vi "Deserialize File Attributes.vi"(8 "error in":errorcluster, 11 "packet":u8[](array[numeric])) -> (0 "error out":errorcluster, 2 "file attributes":T1 {"permissions" format="%04o"}, 3 "packet remaining":u8[](array[numeric]))   [LabVIEW 2020, in "NI_SFTP.lvlib"]
uses:
  <vilib>/net/SFTP/NI_SFTP.lvlib
  <vilib>/net/SFTP/API/Support/File Attributes.ctl
  d022a744-54a9-3fd3-903f-96656418eb3f.vi
  344b3680-f82e-3fd4-783f-4678d93fd33f.vi
  ad0e4a4c-18fc-3fe0-0060-795593d7b03f.vi
  adfa6818-b576-3fe4-a010-b17c7da7e73f.vi
  0b12cbf9-0ffd-3fec-4b35-d5464624ee3f.vi
  d1b708d0-cdb1-3fdd-e8ab-91f32da9d03f.vi
  8c3f788a-5d1b-3fe5-114b-6415c22bea3f.vi
  7090e118-4d07-3fef-a0e5-9088025bb73f.vi
  96fe2671-f19e-3fdc-e0fb-be93fff4e23f.vi
  d13a85d0-f59b-3fbc-06cd-154f57cdda3f.vi
  <vilib>/net/SFTP/Low Level Connection/Assert Length.vi
  <vilib>/Bit Manipulation/Network-Order Bytes To Words Poly.vi
  <vilib>/Bit Manipulation/wrappers/Network-Order Bytes To Words/Network-Order Bytes To Words U32.vi
  <vilib>/Bit Manipulation/wrappers/Network-Order Bytes To Words/Network-Order Bytes To Words U64.vi
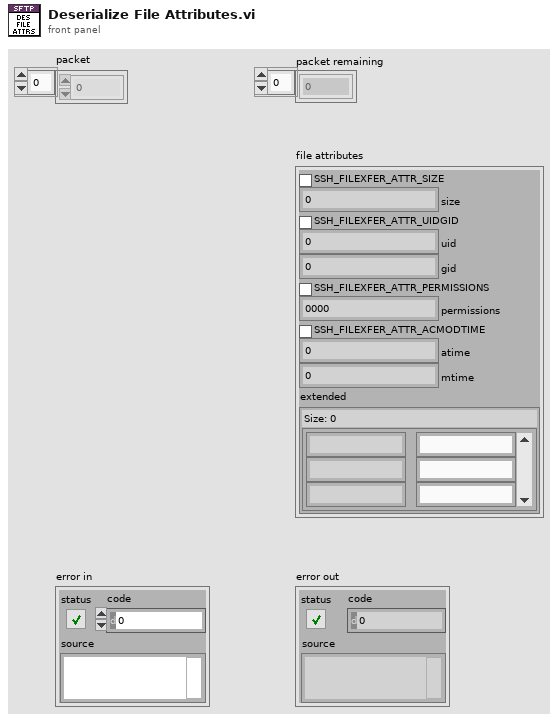
[diagram p1: front panel]
types:
  T1 = typedef "NI_SFTP.lvlib/File Attributes.ctl" = cluster{"SSH_FILEXFER_ATTR_SIZE":bool, "size":u64, "SSH_FILEXFER_ATTR_UIDGID":bool, "uid":u32, "gid":u32, "SSH_FILEXFER_ATTR_PERMISSIONS":bool, "permissions":u32, "SSH_FILEXFER_ATTR_ACMODTIME":bool, "atime":u32, "mtime":u32, "extended":map{string, string}}
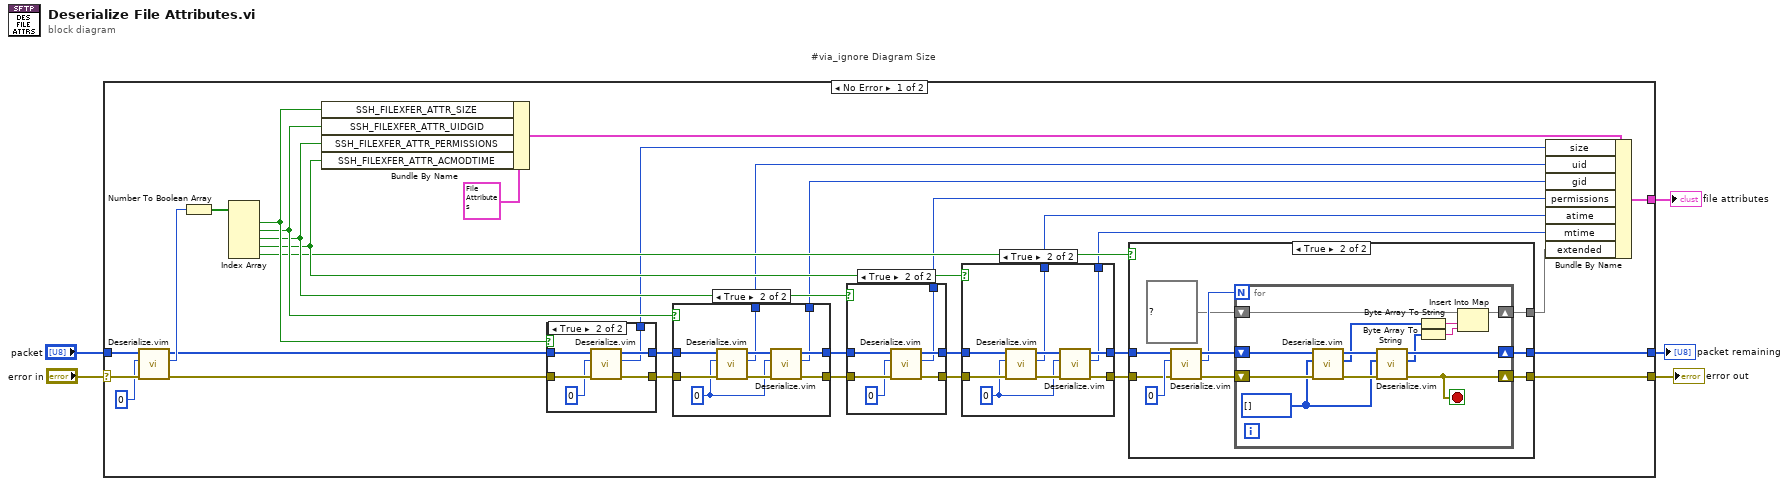
[diagram p0: block diagram]
diagram:
  # "#via_ignore Diagram Size"
  n1 = case shown="No Error" "error in" {
    selector: "error in" -> [w36 w102]
    tunnel: "packet" -> [w37 w101]
    tunnel: [w16 w102] -> w3
    tunnel: [w13 _] -> w2
    tunnel: [w15 w101] -> w1
    frame No Error {
      n2 = call "Deserialize.vim"("error in"=w36, "type"=u32 0, "bytes"=w37) -> ("error out"=w29:errorcluster, "value"=w34:u32, "remaining bytes"=w30:u8[])  [unwired: 6 in]
      n3 = Number To Boolean Array(number=w34) -> (Boolean array=w33:bool[])
      n4 = Index Array(array=w33) -> (element #1=w31:bool, element #2=w28:bool, element #3=w25:bool, element #4=w20:bool, element #5=w19:bool)  [unwired: 5 in]
      n5 = Bundle By Name(cluster=T1 {"SSH_FILEXFER_ATTR_SIZE"=FALSE, "size"=0, "SSH_FILEXFER_ATTR_UIDGID"=FALSE, "uid"=0, "gid"=0, "SSH_FILEXFER_ATTR_PERMISSIONS"=FALSE, "permissions"=0, "SSH_FILEXFER_ATTR_ACMODTIME"=FALSE, "atime"=0, "mtime"=0, "extended"={}} ("File Attributes"), "SSH_FILEXFER_ATTR_SIZE"=w31, "SSH_FILEXFER_ATTR_UIDGID"=w28, "SSH_FILEXFER_ATTR_PERMISSIONS"=w25, "SSH_FILEXFER_ATTR_ACMODTIME"=w20) -> (w6:T1)
      n6 = case shown="True" w31 {
        tunnel: w30 -> [w94 w100]
        tunnel: w29 -> [w93 w99]
        tunnel: [w94 w97] -> w27
        tunnel: [w93 w96] -> w26
        tunnel: [_ w95] -> w7
        frame False {
        }
        frame True {
          n7 = call "Deserialize.vim"("error in"=w99, "type"=u64 0, "bytes"=w100) -> ("error out"=w96:errorcluster, "value"=w95:u64, "remaining bytes"=w97:u8[])  [unwired: 6 in]
        }
      }
      n8 = case shown="True" w28 {
        tunnel: w27 -> [w83 w92]
        tunnel: w26 -> [w82 w91]
        tunnel: [w83 w87] -> w24
        tunnel: [w82 w86] -> w23
        tunnel: [_ w85] -> w9
        tunnel: [_ w84] -> w8
        frame False {
        }
        frame True {
          w88 = u32 0
          n9 = call "Deserialize.vim"("error in"=w91, "type"=w88, "bytes"=w92) -> ("error out"=w89:errorcluster, "value"=w85:u32, "remaining bytes"=w90:u8[])  [unwired: 6 in]
          n10 = call "Deserialize.vim"("error in"=w89, "type"=w88, "bytes"=w90) -> ("error out"=w86:errorcluster, "value"=w84:u32, "remaining bytes"=w87:u8[])  [unwired: 6 in]
        }
      }
      n11 = case shown="True" w25 {
        tunnel: w24 -> [w75 w81]
        tunnel: w23 -> [w74 w80]
        tunnel: [w75 w78] -> w22
        tunnel: [w74 w77] -> w21
        tunnel: [_ w76] -> w10
        frame False {
        }
        frame True {
          n12 = call "Deserialize.vim"("error in"=w80, "type"=u32 0, "bytes"=w81) -> ("error out"=w77:errorcluster, "value"=w76:u32, "remaining bytes"=w78:u8[])  [unwired: 6 in]
        }
      }
      n13 = case shown="True" w20 {
        tunnel: w22 -> [w64 w73]
        tunnel: w21 -> [w63 w72]
        tunnel: [w64 w68] -> w18
        tunnel: [w63 w67] -> w17
        tunnel: [_ w66] -> w12
        tunnel: [_ w65] -> w11
        frame False {
        }
        frame True {
          w69 = u32 0
          n14 = call "Deserialize.vim"("error in"=w72, "type"=w69, "bytes"=w73) -> ("error out"=w70:errorcluster, "value"=w66:u32, "remaining bytes"=w71:u8[])  [unwired: 6 in]
          n15 = call "Deserialize.vim"("error in"=w70, "type"=w69, "bytes"=w71) -> ("error out"=w67:errorcluster, "value"=w65:u32, "remaining bytes"=w68:u8[])  [unwired: 6 in]
        }
      }
      n16 = case shown="True" w19 {
        tunnel: w18 -> [w39 w48]
        tunnel: w17 -> [w38 w47]
        tunnel: [w39 w42] -> w15
        tunnel: [w38 w41] -> w16
        tunnel: [_ w40] -> w14
        frame False {
        }
        frame True {
          n17 = call "Deserialize.vim"("error in"=w47, "type"=u32 0, "bytes"=w48) -> ("error out"=w45:errorcluster, "value"=w44:u32, "remaining bytes"=w46:u8[])  [unwired: 6 in]
          n18 = for {
            N: w44 -> [_]
            shift-right: [w56] -> w42
            shift-left: w46 -> [w62]
            shift-right: [w55] -> w41
            shift-left: w45 -> [w61]
            shift-right: [w57] -> w40
            shift-left: map{string, string} {} ("extended") -> [w58]
            stop <- w55 stop-if-true
            w54 = u8[] [] ("Array")
            n19 = call "Deserialize.vim"("error in"=w61, "type"=w54, "bytes"=w62) -> ("error out"=w59:errorcluster, "value"=w53:u8[], "remaining bytes"=w60:u8[])  [unwired: 6 in]
            n20 = call "Deserialize.vim"("error in"=w59, "type"=w54, "bytes"=w60) -> ("error out"=w55:errorcluster, "value"=w51:u8[], "remaining bytes"=w56:u8[])  [unwired: 6 in]
            n21 = Byte Array To String(unsigned byte array=w53) -> (string=w52:string)
            n22 = Byte Array To String(unsigned byte array=w51) -> (string=w50:string)
            n23 = Insert Into Map(map in=w58, key=w52, value=w50) -> (map out=w57:map{string, string})  [unwired: 2 out]
          }
        }
      }
      n24 = Bundle By Name(cluster=w6, "size"=w7, "uid"=w9, "gid"=w8, "permissions"=w10, "atime"=w12, "mtime"=w11, "extended"=w14) -> (w13:T1)
    }
    frame Error {
    }
  }
  "error out" <- w3
  "file attributes" <- w2
  "packet remaining" <- w1
